vi "String stuff test code with term characterse.vi"() -> ()   [LabVIEW 2015]
panel:
  out "concatenated string":string
  out "Read buffer out":string
  in  "String in":string
  in  "error IO":errorcluster
  in  "stop":bool
  in  "Term Char":string
  out "Read String":string
  out "error out":errorcluster
  in  "error in (no error)":errorcluster
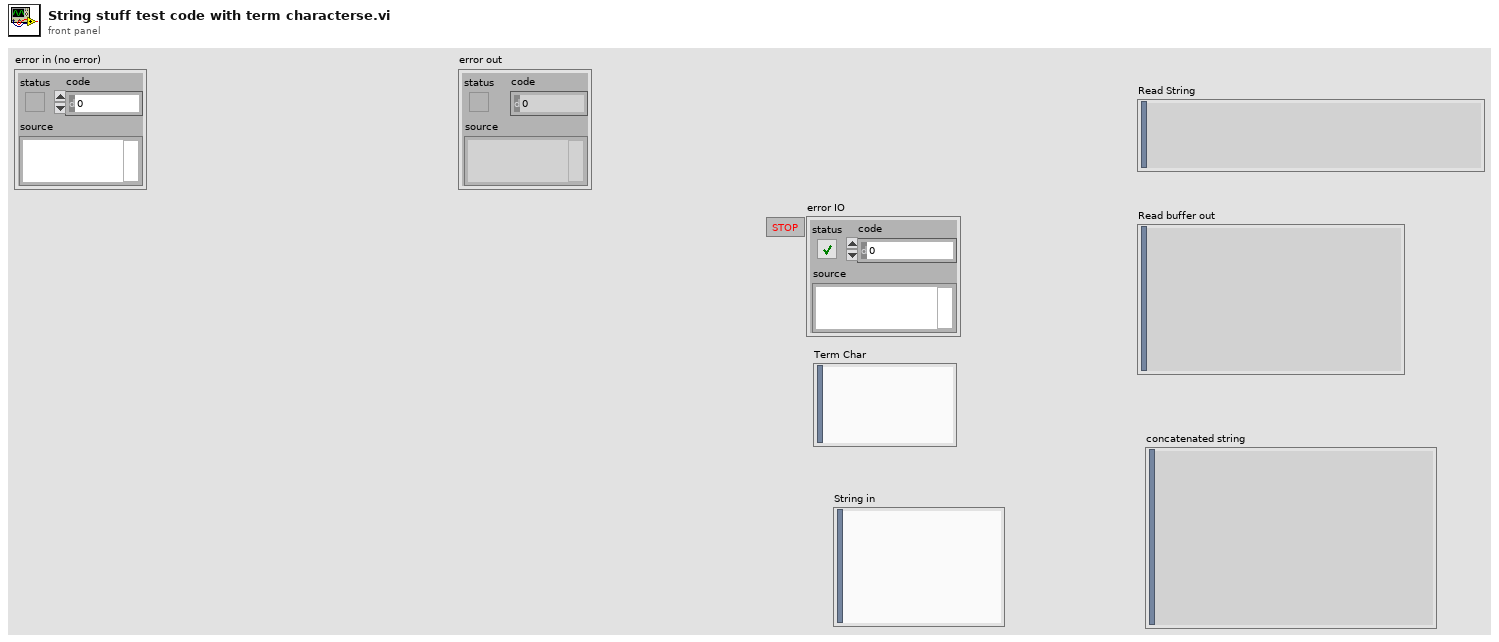
[diagram p1: front panel]
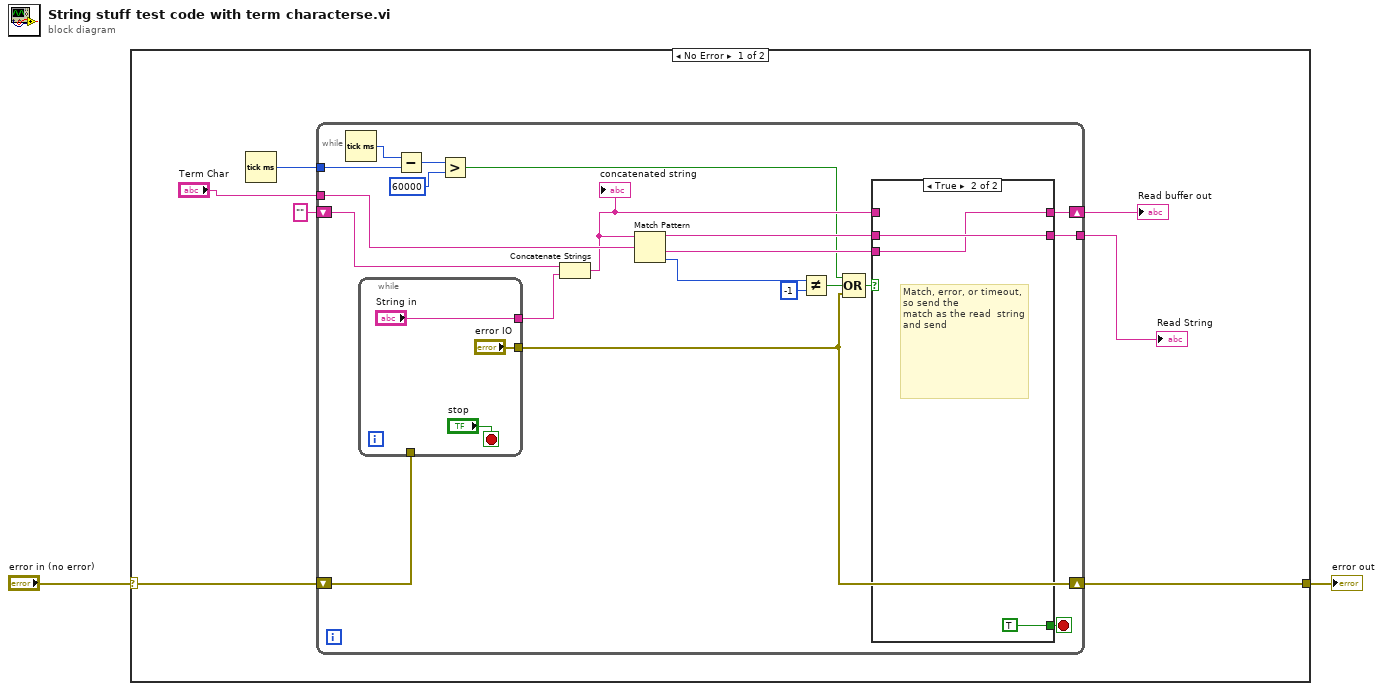
[diagram p0: block diagram]
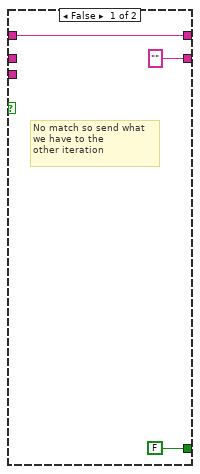
[diagram p2: hidden frame]
diagram:
  n1 = case shown="No Error" "error in (no error)" {
    selector: "error in (no error)" -> [w9 w39]
    tunnel: [w8 w39] -> w1
    frame No Error {
      n2 = Tick Count (ms)() -> (millisecond timer value=w7:u32)
      n3 = while {
        shift-right: [w11] -> w8
        shift-left: w9 -> [w12]
        tunnel: [w23] -> w6
        shift-right: [w22] -> w3
        shift-left: "" -> [w20]
        tunnel: "Term Char" -> [w19]
        tunnel: w7 -> [w17]
        stop <- w24 stop-if-true
        n4 = Tick Count (ms)() -> (millisecond timer value=w16:u32)
        n5 = while {
          tunnel: w12 -> [_]
          tunnel: ["error IO"] -> w11
          tunnel: ["String in"] -> w10
          stop <- "stop" stop-if-true
        }
        n6 = Subtract(x=w16, y=w17) -> (x-y=w15:u32)
        n7 = Greater?(x=w15, y=u32 60000) -> (0:w13:bool)
        n8 = Concatenate Strings(w20, w10) -> (w18:string)
        "concatenated string" <- w18
        n9 = Match Pattern(string=w18, regular expression=w19) -> (before substring=w27:string, after substring=w21:string, offset past match=w29:i32)  [unwired: 1 in, 1 out]
        n10 = Not Equal?(x=w29, y=-1) -> (x != y?=w26:bool)
        n11 = Compound Arithmetic op=OR(w13, w26, w11) -> (w25:bool)
        n12 = case shown="True" w25 {
          tunnel: w27 -> [_ w37]
          tunnel: [FALSE TRUE] -> w24
          tunnel: ["" w37] -> w23
          tunnel: [w34 w36] -> w22
          tunnel: w21 -> [_ w36]
          tunnel: w18 -> [w34 _]
          frame False {
            # "No match so send what\nwe have to the \nother iteration"
          }
          frame True {
            # "Match, error, or timeout, so send the \nmatch as the read  string and send"
          }
        }
      }
      "Read String" <- w6
      "Read buffer out" <- w3
    }
    frame Error {
    }
  }
  "error out" <- w1
